vi "Xbox Layout Cluster.vi"(1 "Joystick Name":string) -> (0 "Joystick Out":T1)   [LabVIEW 2015]
uses:
  <vilib>/Rock Robotics/WPI/Utilities/WPI_GetSetVariantRefNum.vi
panel:
  out "Right Throttle":dbl
  out "Left Throttle":dbl
  out "Arrows":i16
  out "Left Stick Touch":bool
  out "Right Stick Touch":bool
  out "Center Right":bool
  out "Center Left":bool
  out "Right Stick Y":dbl
  out "Right Stick X":dbl
  out "Left Stick Y":dbl
  out "Left Stick X":dbl
  out "X":bool
  out "A":bool
  out "B":bool
  out "Y":bool
  out "Left Button":bool
  out "Right Button":bool
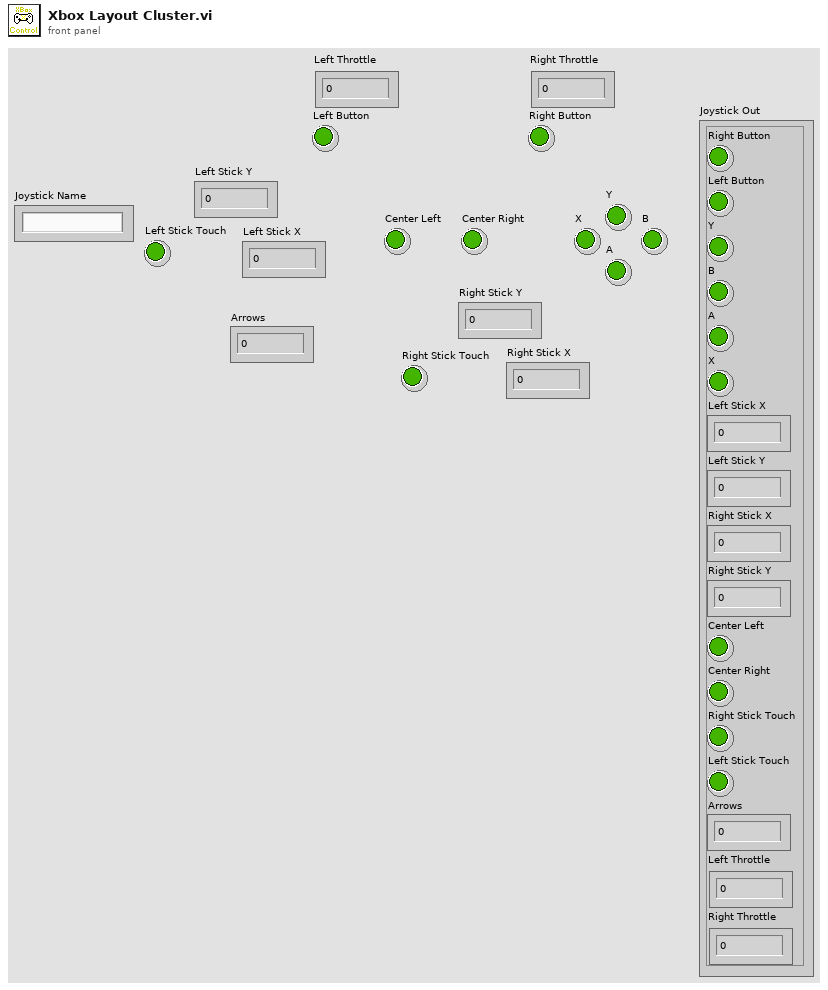
[diagram p1: front panel]
types:
  T1 = cluster{"Right Button":bool, "Left Button ":bool, "Y":bool, "B":bool, "A":bool, "X":bool, "Left Stick X":dbl, "Left Stick Y":dbl, "Right Stick X ":dbl, "Right Stick Y ":dbl, "Center Left":bool, "Center Right":bool, "Right Stick Touch":bool, "Left Stick Touch ":bool, "Arrows":i16, "Left Throttle":dbl, "Right Throttle":dbl}
  T2 = typedef "WPI_JoystickDevRef.ctl" = cluster{"Device":T3}
  T3 = typedef "WPI_JoystickDeviceEnum.ctl" = enum16{"USB 0", "USB 1", "USB 2", "USB 3", "USB 4", "USB 5"}
  T4 = cluster{"Axes[0]":dbl, "Axes[1]":dbl, "Axes[2]":dbl, "Axes[3]":dbl, "Axes[4]":dbl, "Axes[5]":dbl, "Axes[6]":dbl, "Axes[7]":dbl, "Axes[8]":dbl}
  T5 = cluster{"POVs[0]":i16, "POVs[1]":i16, "POVs[2]":i16, "POVs[3]":i16, "POVs[4]":i16, "POVs[5]":i16, "POVs[6]":i16, "POVs[7]":i16, "POVs[8]":i16}
  T6 = cluster{"Button 1":bool, "Button 2":bool, "Button 3":bool, "Button 4":bool, "Button 5":bool, "Button 6":bool, "Button 7":bool, "Button 8":bool, "Button 9":bool, "Button 10":bool, "Button 11":bool, "Button 12":bool}
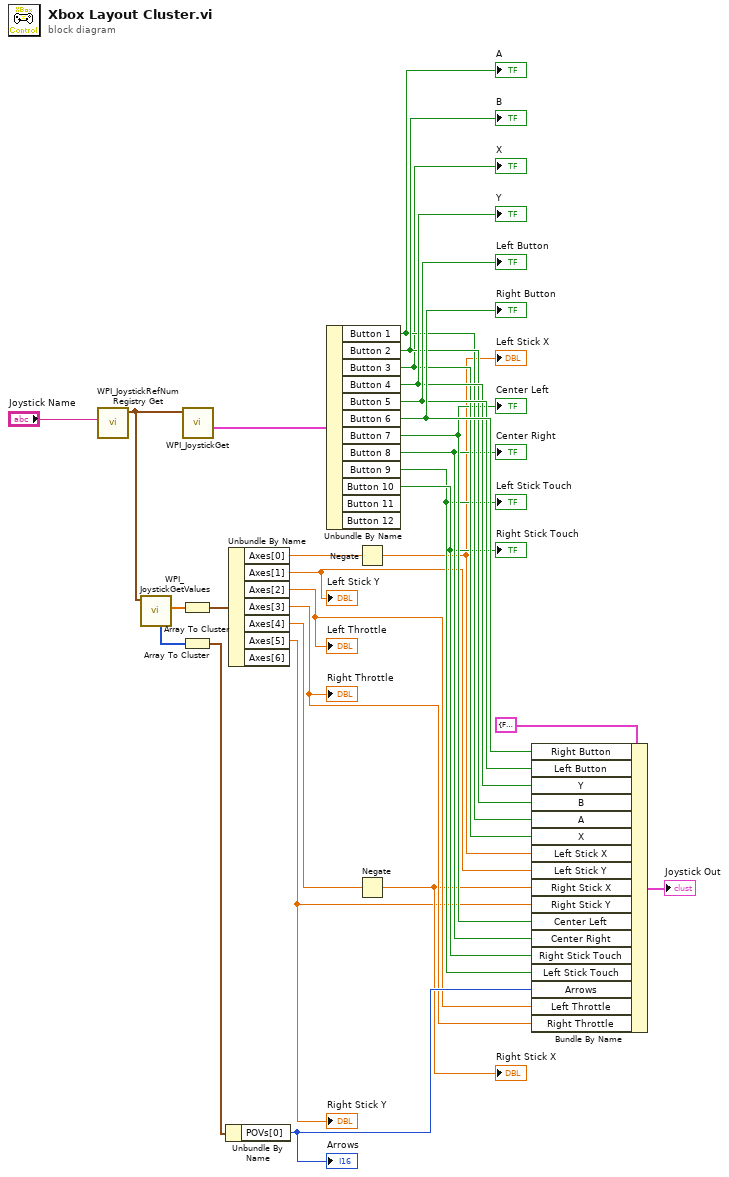
[diagram p0: block diagram]
diagram:
  n1 = call <vilib>:"WPI_JoystickRefNum Registry Get.vi"("refnum name"="Joystick Name") -> ("JoystickDevRef"=w25:T2)  [unwired: 9 in, 1 out]
  n2 = call <vilib>:"WPI_JoystickGetValues.vi"("JoystickDevRef"=w25) -> ("Axes"=w24:dbl[], "POVs"=w21:i16[])  [unwired: 6 in, 3 out]
  n3 = Array To Cluster(array=w24) -> (cluster=w23:T4)
  n4 = Array To Cluster(array=w21) -> (cluster=w20:T5)
  n5 = call <vilib>:"WPI_JoystickGet.vi"("JoystickDevRef"=w25) -> ("Buttons"=w27:T6)  [unwired: 4 in, 2 out]
  n6 = Unbundle By Name(w20) -> ("POVs[0]"=w7:i16)
  "Arrows" <- w7
  n7 = Unbundle By Name(w23) -> ("Axes[0]"=w26:dbl, "Axes[1]"=w3:dbl, "Axes[2]"=w6:dbl, "Axes[3]"=w5:dbl, "Axes[4]"=w22:dbl, "Axes[5]"=w1:dbl)  [unwired: 1 out]
  "Left Stick Y" <- w3
  "Right Stick Y" <- w1
  "Left Throttle" <- w6
  "Right Throttle" <- w5
  n8 = Unbundle By Name(w27) -> ("Button 1"=w13:bool, "Button 2"=w14:bool, "Button 3"=w12:bool, "Button 4"=w15:bool, "Button 5"=w16:bool, "Button 6"=w17:bool, "Button 7"=w11:bool, "Button 8"=w10:bool, "Button 9"=w8:bool, "Button 10"=w9:bool)  [unwired: 2 out]
  "Right Button" <- w17
  "Left Button" <- w16
  "Y" <- w15
  "B" <- w14
  "A" <- w13
  "X" <- w12
  "Center Left" <- w11
  "Center Right" <- w10
  "Right Stick Touch" <- w9
  "Left Stick Touch" <- w8
  n9 = Negate(x=w26) -> (-x=w4:dbl)
  "Left Stick X" <- w4
  n10 = Negate(x=w22) -> (-x=w2:dbl)
  "Right Stick X" <- w2
  n11 = Bundle By Name(cluster=T1 {"Right Button"=FALSE, "Left Button "=FALSE, "Y"=FALSE, "B"=FALSE, "A"=FALSE, "X"=FALSE, "Left Stick X"=0.0, "Left Stick Y"=0.0, "Right Stick X "=0.0, "Right Stick Y "=0.0, "Center Left"=FALSE, "Center Right"=FALSE, "Right Stick Touch"=FALSE, "Left Stick Touch "=FALSE, "Arrows"=0, "Left Throttle"=0.0, "Right Throttle"=0.0} ("Joystick Out 2"), "Right Button"=w17, "Left Button"=w16, "Y"=w15, "B"=w14, "A"=w13, "X"=w12, "Left Stick X"=w4, "Left Stick Y"=w3, "Right Stick X"=w2, "Right Stick Y"=w1, "Center Left"=w11, "Center Right"=w10, "Right Stick Touch"=w9, "Left Stick Touch"=w8, "Arrows"=w7, "Left Throttle"=w6, "Right Throttle"=w5) -> (→"Joystick Out":T1)
